vi "Configure Instrument.vi"(8 "error in (no error)":errorcluster, 11 "VoltageUpdate":refnum<class "VoltageUpdate.lvclass">) -> (0 "error out":errorcluster, 3 "VoltageUpdate out":refnum<class "VoltageUpdate.lvclass">)   [LabVIEW 2016, in "VoltageUpdate.lvclass"]
uses:
  VoltageUpdate.lvclass
  <userlib>/LevyLab/Levylab Instruments/Instrument Types/VSource/Instrument.VSource.lvclass
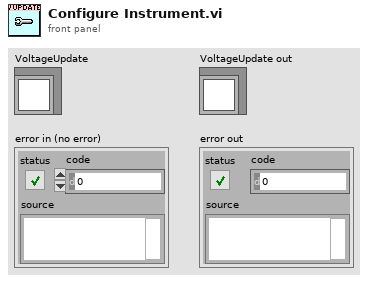
[diagram p1: front panel]
types:
  T1 = typedef "VoltageUpdate.lvclass/VoltageUpdate.Configuration--Cluster.ctl" = cluster{"Amplfier Gain":dbl}
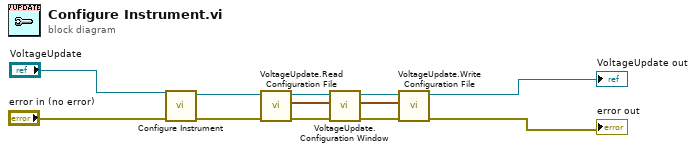
[diagram p0: block diagram]
diagram:
  n1 = call-parent "Configure Instrument.vi"("error in (no error)"="error in (no error)", "Instrument in"="VoltageUpdate") -> ("error out"=w7:errorcluster, "Instrument out"=w9:refnum<class "VoltageUpdate.lvclass">)  [unwired: 8 in]
  n2 = call "VoltageUpdate.Read Configuration File.vi"("error in (no error)"=w7, "VoltageUpdate"=w9) -> ("error out"=w6:errorcluster, "Configuration"=w2:T1, "VoltageUpdate out"=w5:refnum<class "VoltageUpdate.lvclass">)  [unwired: 7 in]
  n3 = call "VoltageUpdate.Configuration Window.vi"("error in (no error)"=w6, "Ex Configuration"=w2, "VoltageUpdate"=w5) -> ("error out"=w3:errorcluster, "output cluster"=w1:T1, "VoltageUpdate out"=w4:refnum<class "VoltageUpdate.lvclass">)  [unwired: 6 in]
  n4 = call "VoltageUpdate.Write Configuration File.vi"("error in (no error)"=w3, "Configuration"=w1, "VoltageUpdate"=w4) -> ("error out"=→"error out":errorcluster, "VoltageUpdate out"=→"VoltageUpdate out":refnum<class "VoltageUpdate.lvclass">)  [unwired: 7 in]
